vi "MHM Get Open Interface.vi"(8 "error in (no error)":errorcluster, 10 "ulInterface":u32, 11 "ulMHMHandle":u32) -> (0 "error out":errorcluster, 3 "ulMHMHandle out":u32)   [LabVIEW 2017]
uses:
  MHM_1SL_interface.lvlib
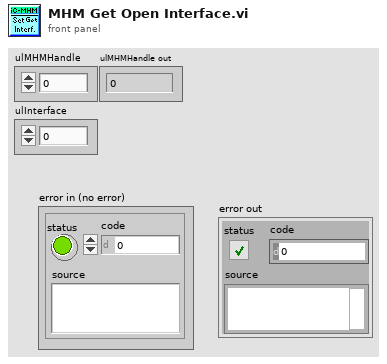
[diagram p1: front panel]
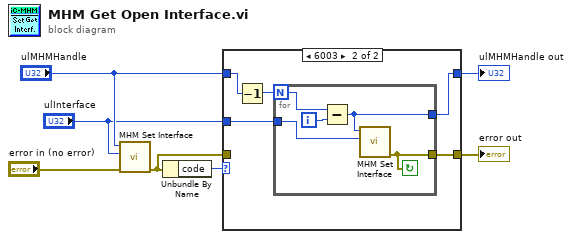
[diagram p0: block diagram]
diagram:
  n1 = call "MHM Set Interface.vi"("error in (no error)"="error in (no error)", "ulInterface"="ulInterface", "ulMHMHandle"="ulMHMHandle") -> ("error out"=w2:errorcluster)  [unwired: 7 in, 1 out]
  n2 = Unbundle By Name(w2) -> ("code"=w7:i32)
  n3 = case shown="6003" w7 {
    tunnel: "ulMHMHandle" -> [w9 w13]
    tunnel: "ulInterface" -> [_ w12]
    tunnel: [w9 w11] -> w4
    tunnel: w2 -> [w8 _]
    tunnel: [w8 w10] -> w1
    frame 0, Default {
    }
    frame 6003 {
      n4 = Decrement(x=w13) -> (x-1=w14:u32)
      n5 = for {
        N: w14 -> [w18]
        tunnel: w12 -> [w17]
        tunnel: [w16] -> w11
        tunnel: [w15] -> w10
        i -> [w19]
        stop <- w15 continue-if-true
        n6 = Subtract(x=w18, y=w19) -> (x-y=w16:i32)
        n7 = call "MHM Set Interface.vi"("ulInterface"=w17, "ulMHMHandle"=w16) -> ("error out"=w15:errorcluster)  [unwired: 8 in, 1 out]
      }
    }
  }
  "ulMHMHandle out" <- w4
  "error out" <- w1
